vi "VI Server_MenuRing_Update_ItemNames_FromSpeadsheetString.vi"(6 "Strings []: SpreadsheetFormat":string, 7 "Label":string, 8 "error in":errorcluster, 11 "VI Server Cluster":T1) -> (0 "error out":errorcluster, 1 "Control Reference":refnum<vi>, 3 "VI Server Cluster.DUP":T1, 4 "ItemNames":string[](array[string]))   [LabVIEW 2020, in "VI Server Toolkit LV2013.lvlib"]
doc: "Updates Menu Ring Items List from spreadsheet string (comma-delimited)."
uses:
  VI Server Toolkit LV2013.lvlib
  VI Server_TypeDefs/VI Server_RefsCluster.ctl
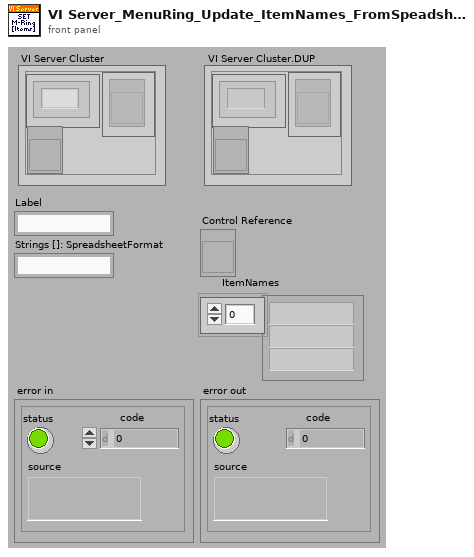
[diagram p1: front panel]
types:
  T1 = typedef "VI Server_RefsCluster.ctl" = cluster{"Labels":string[], "Refs":refnum<vi>[], "VI Ref":refnum<vi>}
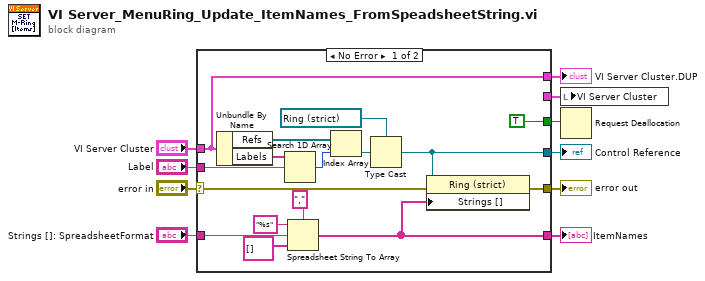
[diagram p0: block diagram]
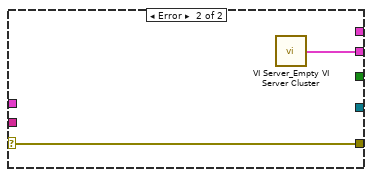
[diagram p2: hidden frame]
diagram:
  n1 = case shown="No Error" "error in" {
    selector: "error in" -> [w21 w28]
    tunnel: "Label" -> [w25 _]
    tunnel: "VI Server Cluster" -> [w13 _]
    tunnel: [w20 w28] -> w10
    tunnel: [w19 _] -> w6
    tunnel: "Strings []: SpreadsheetFormat" -> [w18 _]
    tunnel: [w13 _] -> w4
    tunnel: [TRUE _] -> w3
    tunnel: [_ w27] -> w2
    tunnel: [w11 _] -> w1
    frame No Error {
      n2 = Unbundle By Name(w13) -> ("Refs"=w23:refnum<vi>[], "Labels"=w26:string[])
      n3 = Search 1D Array(1D array=w26, element=w25) -> (index of element=w24:i32)  [unwired: 1 out]
      n4 = Spreadsheet String To Array(delimiter (Tab)=",", format string="%s", spreadsheet string=w18, array type (2D Dbl)=string[] []) -> (array=w11:string[])
      n5 = Index Array(array=w23, index=w24) -> (element=w22:refnum<vi>)
      n6 = Type Cast(type=refnum<vi> refnum ("Ring"), x=w22) -> (*(type *) &x=w19:refnum<vi>)
      n7 = property class="Ring (strict)"(reference=w19, error in=w21, "Strings []"=w11) -> (error out=w20:errorcluster)  [unwired: 1 out]
    }
    frame Error {
      n8 = call "VI Server_Empty VI Server Cluster.vi"() -> ("VI Server Cluster"=w27:T1)  [unwired: 7 in]
    }
  }
  "error out" <- w10
  "VI Server Cluster.DUP" <- w4
  "Control Reference" <- w6
  "ItemNames" <- w1
  n9 = local write "VI Server Cluster"(w2) -> ()
  n10 = Request Deallocation(w3) -> ()
